vi "Write Running Measurements Lookup Table.vi"(8 "error in (no error)":errorcluster, 10 "Running Measurements Lookup Table":variant, 11 "Controller in":refnum<class "Controller.lvclass">) -> (0 "error out":errorcluster, 3 "Controller out":refnum<class "Controller.lvclass">)   [LabVIEW 2015, in "Controller Actor.lvlib" / "Controller.lvclass"]
uses:
  Controller.lvclass
  Controller.lvclass/Controller.ctl
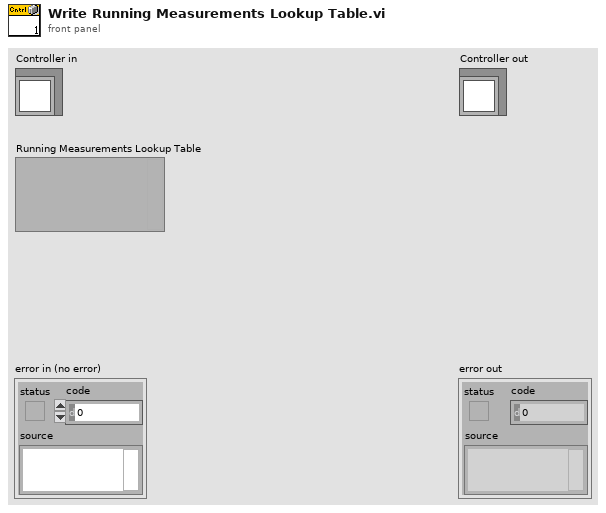
[diagram p1: front panel]
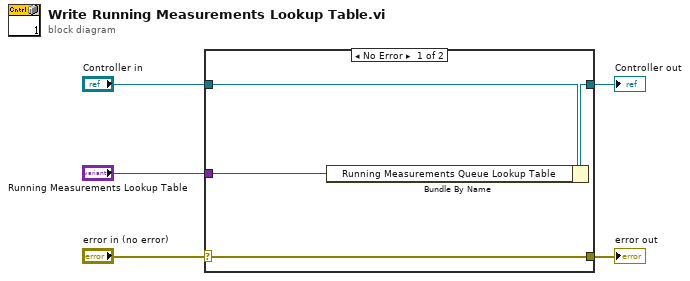
[diagram p0: block diagram]
diagram:
  n1 = case shown="No Error" "error in (no error)" {
    selector: "error in (no error)" -> [w9 w10]
    tunnel: [w9 w10] -> w4
    tunnel: [w7 w11] -> w2
    tunnel: "Controller in" -> [w8 w11]
    tunnel: "Running Measurements Lookup Table" -> [w6 _]
    frame No Error {
      n2 = Bundle By Name(cluster=w8, "Running Measurements Queue Lookup Table"=w6) -> (w7:refnum<class "Controller.lvclass">)
    }
    frame Error {
    }
  }
  "error out" <- w4
  "Controller out" <- w2
